vi "Generate Worker Info.vi"(8 "error in (no error)":errorcluster, 11 "Worker lvlib":path) -> (0 "error out":errorcluster, 1 "Icon":T2, 2 "Special Terminals":T1={"Action"=-1, "Init"=-1, "Tag"=-1, "State in"=-1, "State out"=-1, "Error"=-1}, 3 "Type Descriptors":T3[](array[typedef]))   [LabVIEW 2020, in "FlexBlocks.lvlib"]
uses:
  FlexBlocks.lvlib
  Type Descriptor.ctl
  Terminal Direction.ctl
  Value Mode.ctl
  Special Terminal.ctl
  <vilib>/picture/picture.llb/imagedata.ctl
  Special Terminal Indices.ctl
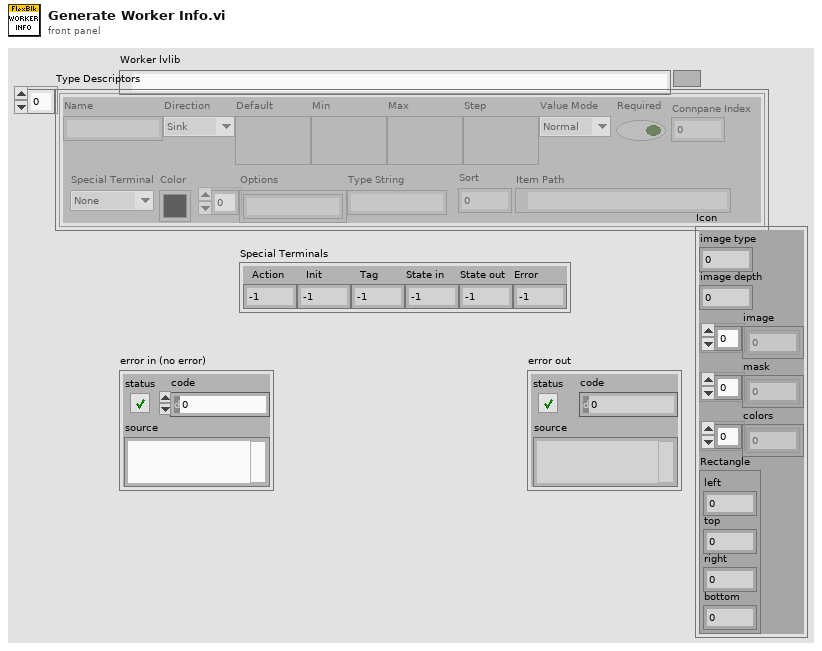
[diagram p1: front panel]
types:
  T1 = typedef "FlexBlocks.lvlib/Special Terminal Indices.ctl" = cluster{"Action":i32, "Init":i32, "Tag":i32, "State in":i32, "State out":i32, "Error":i32}
  T2 = typedef "imagedata.ctl" = cluster{"image type":i32, "image depth":i32, "image":u8[], "mask":u8[], "colors":u32[], "Rectangle":cluster{"left":i16, "top":i16, "right":i16, "bottom":i16}}
  T3 = typedef "FlexBlocks.lvlib/Type Descriptor.ctl" = cluster{"Name":string, "Direction":T4, "Default":variant, "Min":variant, "Max":variant, "Step":variant, "Value Mode":T5, "Required":bool, "Connpane Index":i32, "Special Terminal":T6, "Color":u32, "Options":string[], "Type String":string, "Sort":i32, "Item Path":path}
  T4 = typedef "FlexBlocks.lvlib/Terminal Direction.ctl" = enum16{"Sink", "Source"}
  T5 = typedef "FlexBlocks.lvlib/Value Mode.ctl" = enum16{"Normal", "Range", "Select"}
  T6 = typedef "FlexBlocks.lvlib/Special Terminal.ctl" = enum16{"None", "Action", "Init", "Tag", "State in", "State out", "Error"}
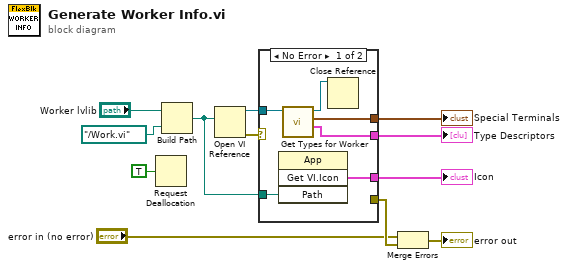
[diagram p0: block diagram]
diagram:
  n1 = Request Deallocation(TRUE ("flag")) -> ()
  n2 = Build Path(base path="Worker lvlib", name or relative path=path "../Work.vi") -> (appended path=w10:path)
  n3 = Open VI Reference(vi path=w10) -> (vi reference=w9:refnum<vi>, error out=w5:errorcluster)  [unwired: 5 in]
  n4 = case shown="No Error" w5 {
    selector: w5 -> [_ w19]
    tunnel: w10 -> [w18 _]
    tunnel: w9 -> [w17 _]
    tunnel: [w16 _] -> w8
    tunnel: [w15 _] -> w7
    tunnel: [w14 _] -> w6
    tunnel: [_ w19] -> w4
    frame No Error {
      n5 = invoke class="App" method="Get VI.Icon"("Path"=w18) -> ("Get VI.Icon"=w16:T2)  [unwired: 3 in, 3 out]
      n6 = call "Get Types for Worker.vi"("Worker VI In"=w17) -> ("Types"=w15:T3[], "Special Terminals"=w14:T1, "Worker VI"=w13:refnum<vi>)  [unwired: 8 in]
      n7 = Close Reference(reference=w13) -> ()  [unwired: 1 in, 1 out]
    }
    frame Error {
    }
  }
  "Type Descriptors" <- w7
  "Icon" <- w8
  "Special Terminals" <- w6
  n8 = Merge Errors("error in (no error)", w4) -> (→"error out":errorcluster)
